vi "RTS Find Opening Order.vi"(7 "Current Status":string[](array[string]), 11 "Selected Order":enum16{"", "1st", "2nd", "3rd"}[](array[ring])) -> (1 "Current Status Output":string[](array[string]), 2 "Run Order":u8[](array[numeric]), 3 "Array Size":i32)   [LabVIEW 2016]
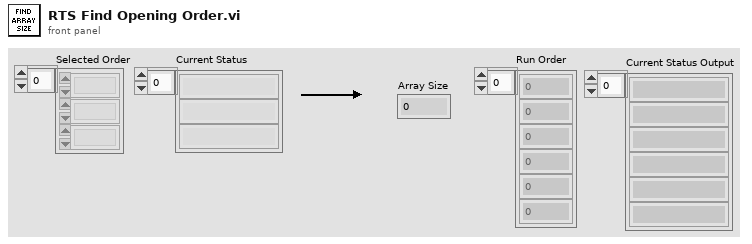
[diagram p1: front panel]
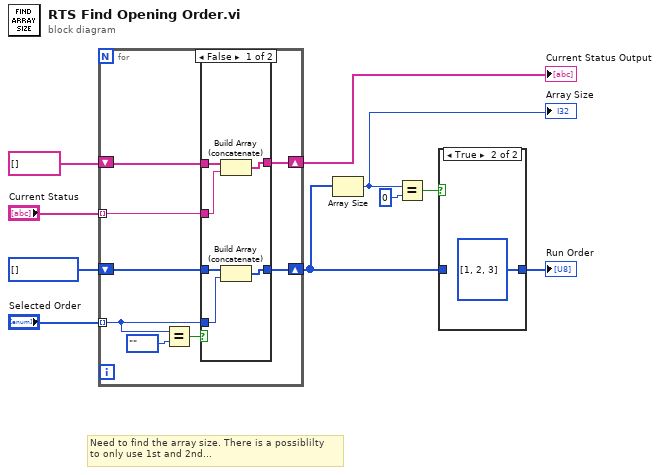
[diagram p0: block diagram]
diagram:
  w9 = enum16{"", "1st", "2nd", "3rd"}[] [] items=["", "1st", "2nd", "3rd"]
  # "Need to find the array size. There is a possiblilty \nto only use 1st and 2nd..."
  n1 = for {
    tunnel: "Selected Order" -> [w16] mode=indexing
    shift-right: [w15] -> w4
    shift-left: w9 -> [w14]
    tunnel: "Current Status" -> [w11] mode=indexing
    shift-right: [w12] -> w1
    shift-left: string[] [] -> [w13]
    n2 = Equal?(x=w16, y=enum16{"", "1st", "2nd", "3rd"}."") -> (x = y?=w17:bool)
    n3 = case shown="False" w17 {
      tunnel: w16 -> [w24 _]
      tunnel: [w23 w26] -> w15
      tunnel: w14 -> [w22 w26]
      tunnel: w13 -> [w21 w25]
      tunnel: [w20 w25] -> w12
      tunnel: w11 -> [w19 _]
      frame False {
        n4 = Build Array (concatenate)(w21, w19) -> (w20:string[])
        n5 = Build Array (concatenate)(w22, w24) -> (w23:enum16{"", "1st", "2nd", "3rd"}[])
      }
      frame True {
      }
    }
  }
  "Current Status Output" <- w1
  n6 = Array Size(array=w4) -> (size(s)=w8:i32)
  "Array Size" <- w8
  n7 = Equal?(x=w8, y=0) -> (x = y?=w6:bool)
  n8 = case shown="True" w6 {
    tunnel: [w27 u8[] [1, 2, 3] ("Run Order 2")] -> w5
    tunnel: w4 -> [w27 _]
    frame False {
    }
    frame True {
    }
  }
  "Run Order" <- w5
